vi "Server.vi"() -> ()   [LabVIEW 2015]
panel:
  out "error out":errorcluster
  out "success 2":u16
  out "success":u16
  out "Data Recv":string
  in  "Data Send":string="Test data server"
  in  "IPv6 Port":dbl=1050.0
  in  "IPv6 Address":string="2001:0DB8:AC10:FE01:0000:0000:0000:0000"
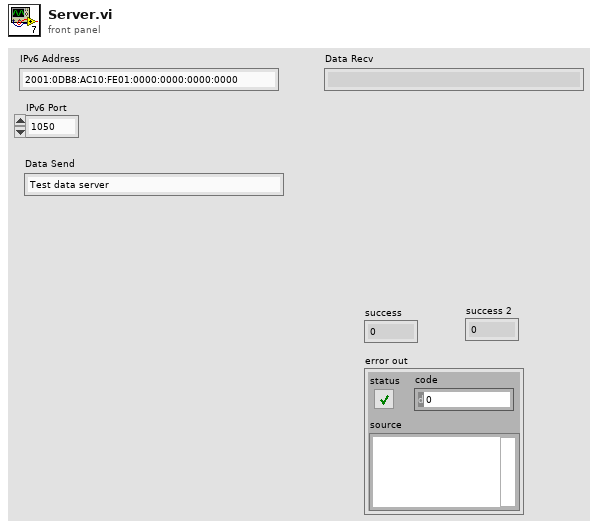
[diagram p1: front panel]
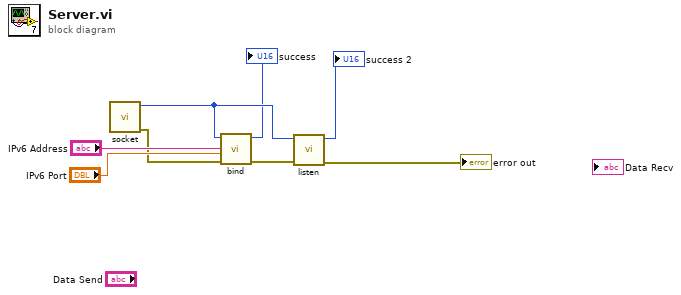
[diagram p0: block diagram]
diagram:
  n1 = call "socket.vi"() -> ("error out"=w6:errorcluster, "tcp socket fd"=w4:i32)  [unwired: 10 in]
  n2 = call "bind.vi"("error in (no error)"=w6, "sin6_port"="IPv6 Port", "sin6_addr"="IPv6 Address", "tcp socket fd"=w4) -> ("error out"=w5:errorcluster, "success"=→"success":u16)  [unwired: 6 in]
  n3 = call "listen.vi"("error in (no error)"=w5, "tcp socket fd"=w4) -> ("error out"=→"error out":errorcluster, "success"=→"success 2":u16)  [unwired: 8 in]
